vi "IFD Img Info mk2.vi"(8 "error in (no error)":errorcluster, 9 "Data type":T1, 10 "size(s)":i32[](array[numeric]), 11 "IFD in":refnum<class "IFD.lvclass">) -> (0 "error out":errorcluster, 3 "IFD out":refnum<class "IFD.lvclass">)   [LabVIEW 2016, in "IFD.lvclass"]
uses:
  IFD.lvclass
  Img Data Type.ctl
  IFD.lvclass/IFD.ctl
  Tag/IFD_Tag.lvclass/IFD_Tag.ctl
  Tag/IFD_Tag.lvclass
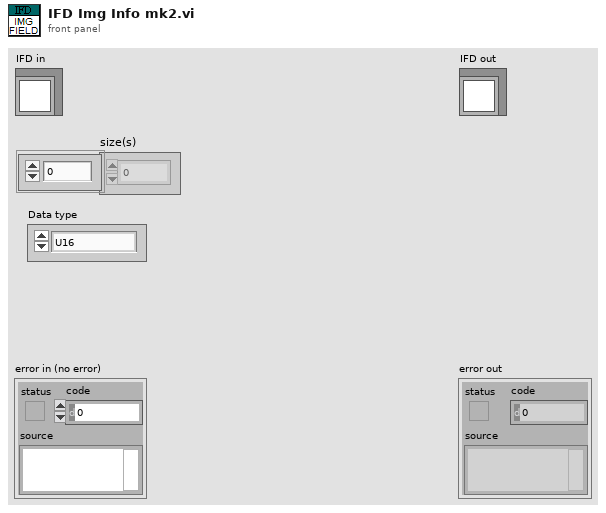
[diagram p1: front panel]
types:
  T1 = typedef "Img Data Type.ctl" = enum16{"U16", "RGB", "SGL"}
  T2 = enum16{"big-endian, network order", "native, host order", "little-endian"}
  T3 = enum16{"Undefined(DO NOT USE)", "U8", "ASCII", "U16", "U32", "RATIONAL", "I8", "Undefined 8 bit", "I16", "I32", "SRATIONAL", "SGL", "DBL"}
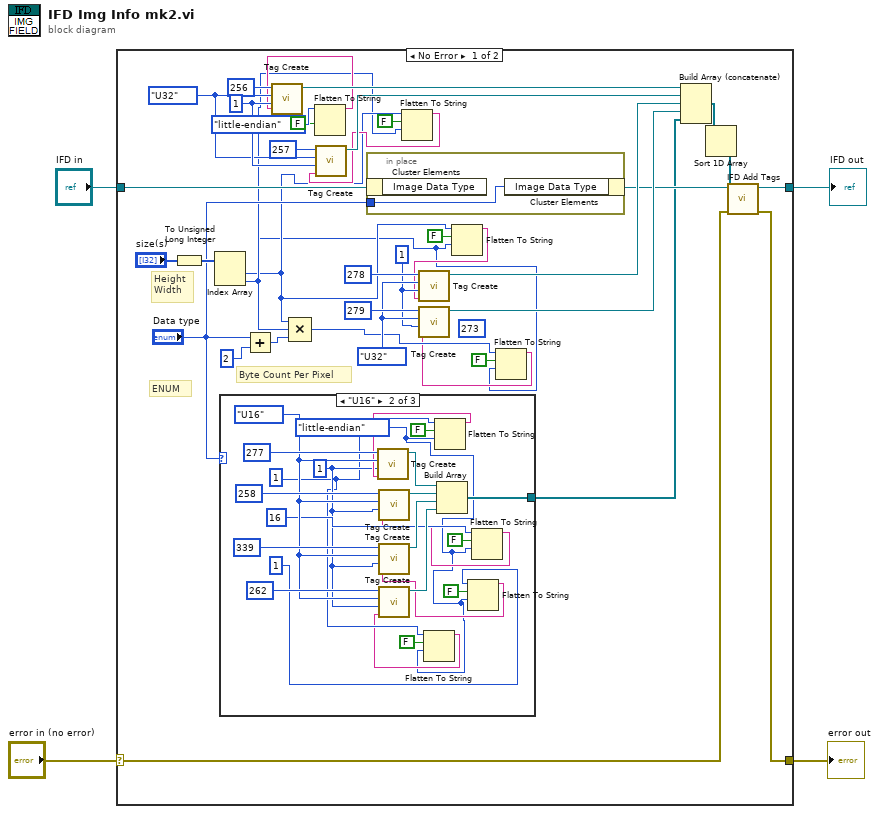
[diagram p0: block diagram]
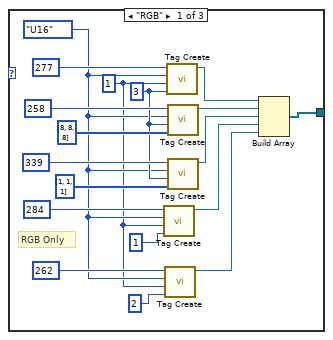
[diagram p2: hidden frame]
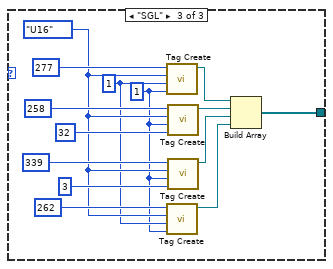
[diagram p3: hidden frame]
diagram:
  n1 = case shown="No Error" "error in (no error)" {
    selector: "error in (no error)" -> [w28 w99]
    tunnel: [w27 w99] -> w3
    tunnel: [w25 w98] -> w1
    tunnel: "IFD in" -> [w26 w98]
    frame No Error {
      w5 = T2."little-endian" ("byte order (0:big-endian, network order)")
      (unwired) u16 273 ("Tag ID")
      w19 = u32 1 ("Data Count")
      w20 = T3."U32" ("Data Type")
      w39 = u32 1 ("Data Count")
      w38 = T3."U32" ("Data Type")
      # "ENUM"
      # "Byte Count Per Pixel"
      # "Height\nWidth"
      n2 = To Unsigned Long Integer(number="size(s)") -> (unsigned 32bit integer=w35:u32[])
      n3 = Index Array(array=w35) -> (element #1=w10:u32, element #2=w16:u32)  [unwired: 2 in]
      n4 = case shown="\"U16\"" "Data type" {
        tunnel: [w48 w77 w89] -> w18
        frame "RGB" {
          w55 = u16 3
          w45 = u32 1 ("Data Count")
          w46 = T3."U16" ("Data Type")
          # "RGB Only"
          n5 = call "Tag Create.vi"("Data"=u16 1, "Data Count"=w45, "Data Type"=w46, "Tag ID"=u16 284) -> ("IFD_Tag out"=w49:refnum<class "IFD_Tag.lvclass">)  [unwired: 7 in]
          n6 = call "Tag Create.vi"("Data"=u16 2, "Data Count"=w45, "Data Type"=w46, "Tag ID"=u16 262) -> ("IFD_Tag out"=w43:refnum<class "IFD_Tag.lvclass">)  [unwired: 7 in]
          n7 = call "Tag Create.vi"("Data"=w55, "Data Count"=w45, "Data Type"=w46, "Tag ID"=u16 277) -> ("IFD_Tag out"=w52:refnum<class "IFD_Tag.lvclass">)  [unwired: 7 in]
          n8 = call "Tag Create.vi"("Data"=u16[] [8, 8, 8], "Data Count"=w55, "Data Type"=w46, "Tag ID"=u16 258) -> ("IFD_Tag out"=w51:refnum<class "IFD_Tag.lvclass">)  [unwired: 7 in]
          n9 = call "Tag Create.vi"("Data"=u16[] [1, 1, 1], "Data Count"=w55, "Data Type"=w46, "Tag ID"=u16 339) -> ("IFD_Tag out"=w50:refnum<class "IFD_Tag.lvclass">)  [unwired: 7 in]
          n10 = Build Array(w52, w51, w50, w49, w43) -> (w48:refnum<class "IFD_Tag.lvclass">[])
        }
        frame "U16" {
          w62 = T2."little-endian" ("byte order (0:big-endian, network order)")
          w64 = u16 1
          w67 = u32 1 ("Data Count")
          w74 = T3."U16" ("Data Type")
          n11 = Flatten To String(anything=w64, prepend array or string size? (T)=FALSE, byte order (0:big-endian, network order)=w62) -> (data string=w63:string)  [unwired: 1 in, 2 out]
          n12 = call "Tag Create.vi"("Data"=w63, "Data Count"=w67, "Data Type"=w74, "Tag ID"=u16 262) -> ("IFD_Tag out"=w75:refnum<class "IFD_Tag.lvclass">)  [unwired: 7 in]
          n13 = Flatten To String(anything=w64, prepend array or string size? (T)=FALSE, byte order (0:big-endian, network order)=w62) -> (data string=w72:string)  [unwired: 1 in, 2 out]
          n14 = call "Tag Create.vi"("Data"=w72, "Data Count"=w67, "Data Type"=w74, "Tag ID"=u16 277) -> ("IFD_Tag out"=w80:refnum<class "IFD_Tag.lvclass">)  [unwired: 7 in]
          n15 = Flatten To String(anything=u16 1, prepend array or string size? (T)=FALSE, byte order (0:big-endian, network order)=w62) -> (data string=w66:string)  [unwired: 1 in, 2 out]
          n16 = call "Tag Create.vi"("Data"=w66, "Data Count"=w67, "Data Type"=w74, "Tag ID"=u16 339) -> ("IFD_Tag out"=w78:refnum<class "IFD_Tag.lvclass">)  [unwired: 7 in]
          n17 = Flatten To String(anything=u16 16, prepend array or string size? (T)=FALSE, byte order (0:big-endian, network order)=w62) -> (data string=w69:string)  [unwired: 1 in, 2 out]
          n18 = call "Tag Create.vi"("Data"=w69, "Data Count"=w67, "Data Type"=w74, "Tag ID"=u16 258) -> ("IFD_Tag out"=w79:refnum<class "IFD_Tag.lvclass">)  [unwired: 7 in]
          n19 = Build Array(w80, w79, w78, w75) -> (w77:refnum<class "IFD_Tag.lvclass">[])
        }
        frame "SGL" {
          w84 = u16 1
          w85 = u32 1 ("Data Count")
          w86 = T3."U16" ("Data Type")
          n20 = call "Tag Create.vi"("Data"=w84, "Data Count"=w85, "Data Type"=w86, "Tag ID"=u16 277) -> ("IFD_Tag out"=w92:refnum<class "IFD_Tag.lvclass">)  [unwired: 7 in]
          n21 = call "Tag Create.vi"("Data"=w84, "Data Count"=w85, "Data Type"=w86, "Tag ID"=u16 262) -> ("IFD_Tag out"=w87:refnum<class "IFD_Tag.lvclass">)  [unwired: 7 in]
          n22 = call "Tag Create.vi"("Data"=u16 32, "Data Count"=w84, "Data Type"=w86, "Tag ID"=u16 258) -> ("IFD_Tag out"=w91:refnum<class "IFD_Tag.lvclass">)  [unwired: 7 in]
          n23 = call "Tag Create.vi"("Data"=u16 3, "Data Count"=w84, "Data Type"=w86, "Tag ID"=u16 339) -> ("IFD_Tag out"=w90:refnum<class "IFD_Tag.lvclass">)  [unwired: 7 in]
          n24 = Build Array(w92, w91, w90, w87) -> (w89:refnum<class "IFD_Tag.lvclass">[])
        }
      }
      n25 = Add(x="Data type", y=u32 2) -> (x+y=w21:u32)
      n26 = Compound Arithmetic op=MULTIPLY(w10, w16, w21) -> (w7:u32)
      n27 = Flatten To String(anything=w16, prepend array or string size? (T)=FALSE, byte order (0:big-endian, network order)=w5) -> (data string=w15:string)  [unwired: 1 in, 2 out]
      n28 = call "Tag Create.vi"("Data"=w15, "Data Count"=w39, "Data Type"=w38, "Tag ID"=u16 256) -> ("IFD_Tag out"=w22:refnum<class "IFD_Tag.lvclass">)  [unwired: 7 in]
      n29 = in-place {
        in-place-border: "Data type" -> [w42]
        n30 = in-place-cluster #1(w26) -> ()  [unwired: 1 out]
        n31 = in-place-cluster #1("Image Data Type"=w42) -> (w30:refnum<class "IFD.lvclass">)
      }
      n32 = Flatten To String(anything=w10, prepend array or string size? (T)=FALSE, byte order (0:big-endian, network order)=w5) -> (data string=w13:string)  [unwired: 1 in, 2 out]
      n33 = call "Tag Create.vi"("Data"=w13, "Data Count"=w39, "Data Type"=w38, "Tag ID"=u16 257) -> ("IFD_Tag out"=w23:refnum<class "IFD_Tag.lvclass">)  [unwired: 7 in]
      n34 = Flatten To String(anything=w10, prepend array or string size? (T)=FALSE, byte order (0:big-endian, network order)=w5) -> (data string=w9:string)  [unwired: 1 in, 2 out]
      n35 = call "Tag Create.vi"("Data"=w9, "Data Count"=w19, "Data Type"=w20, "Tag ID"=u16 278) -> ("IFD_Tag out"=w33:refnum<class "IFD_Tag.lvclass">)  [unwired: 7 in]
      n36 = Flatten To String(anything=w7, prepend array or string size? (T)=FALSE, byte order (0:big-endian, network order)=w5) -> (data string=w6:string)  [unwired: 1 in, 2 out]
      n37 = call "Tag Create.vi"("Data"=w6, "Data Count"=w19, "Data Type"=w20, "Tag ID"=u16 279) -> ("IFD_Tag out"=w31:refnum<class "IFD_Tag.lvclass">)  [unwired: 7 in]
      n38 = Build Array (concatenate)(w22, w23, w33, w31, w18) -> (w24:refnum<class "IFD_Tag.lvclass">[])
      n39 = Sort 1D Array(array=w24) -> (sorted array=w17:refnum<class "IFD_Tag.lvclass">[])
      n40 = call "IFD Add Tags.vi"("error in (no error)"=w28, "Tag(s)"=w17, "IFD in"=w30) -> ("error out"=w27:errorcluster, "IFD out"=w25:refnum<class "IFD.lvclass">)  [unwired: 7 in]
    }
    frame Error {
    }
  }
  "error out" <- w3
  "IFD out" <- w1
